vi "New Timed Average Buffer.vi"(9 "Buffer Duration [s]":dbl=1.0, 11 "TimedBuffer in":refnum<class "TimedAverageBuffer.lvclass">) -> (0 "error out":errorcluster, 3 "Timed Average Buffer":T1)   [LabVIEW 2015, in "TimedAverageBuffer.lvlib" / "TimedAverageBuffer.lvclass"]
uses:
  TimedAverageBuffer.lvclass
  TimedAverageBuffer Reference.ctl
  TimedAverageBuffer.lvclass/TimedAverageBuffer.ctl
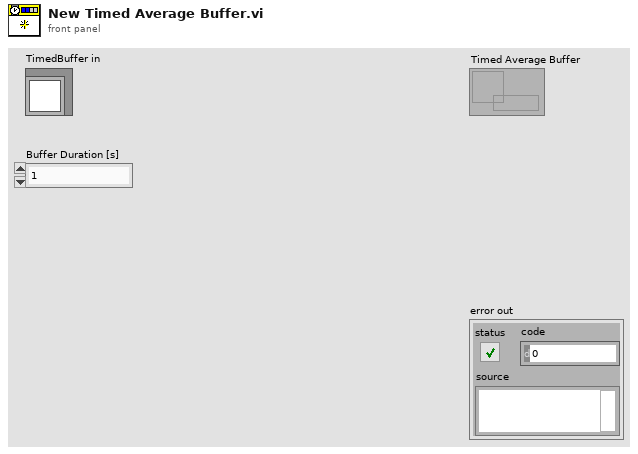
[diagram p1: front panel]
types:
  T1 = typedef "TimedAverageBuffer.lvlib/TimedAverageBuffer.lvclass/TimedAverageBuffer Reference.ctl" = refnum<data-value>
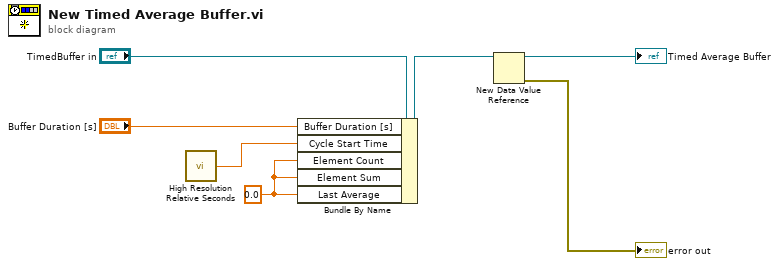
[diagram p0: block diagram]
diagram:
  w3 = 0.0 ("Last Average")
  n1 = call <vilib>:"High Resolution Relative Seconds.vi"() -> ("relative seconds"=w2:dbl)
  n2 = Bundle By Name(cluster="TimedBuffer in", "Buffer Duration [s]"="Buffer Duration [s]", "Cycle Start Time"=w2, "Element Count"=w3, "Element Sum"=w3, "Last Average"=w3) -> (w6:refnum<class "TimedAverageBuffer.lvclass">)
  n3 = New Data Value Reference(data value=w6) -> (data value reference=→"Timed Average Buffer":refnum<data-value>, error out=→"error out":errorcluster)  [unwired: 1 in]
